vi "模拟量输入自动测试.vi"(8 "AD选择?":bool, 10 "DSP选择?":bool) -> ()   [LabVIEW 2010]
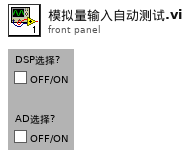
[diagram p1: front panel]
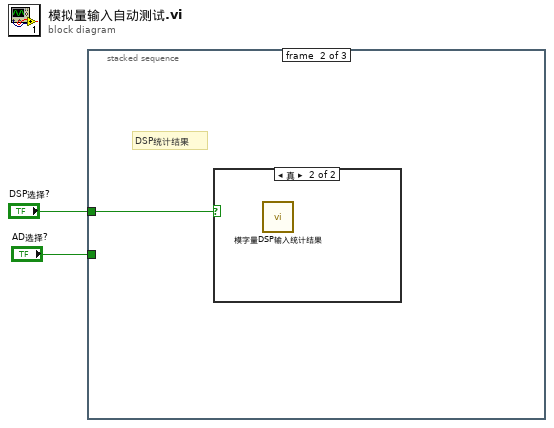
[diagram p0: block diagram]
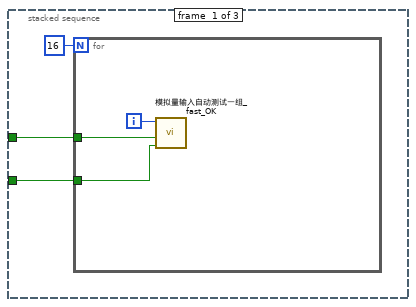
[diagram p2: hidden frame]
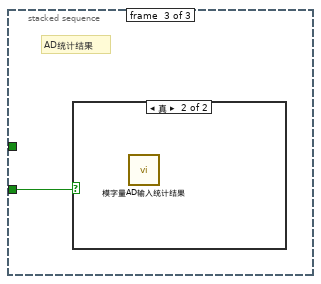
[diagram p4: hidden frame]
diagram:
  n1 = stacked-sequence {
    tunnel: "DSP选择?" -> [w4 w9 _]
    tunnel: "AD选择?" -> [w3 _ w10]
    frame #0 {
      n2 = for {
        N: 16 -> [_]
        tunnel: w4 -> [w7]
        tunnel: w3 -> [w6]
        i -> [w8]
        n3 = call "模拟量输入自动测试一组_fast_OK.vi"("AD选择？"=w6, "DSP选择？"=w7, "第几个"=w8) -> ()  [unwired: 9 in]
      }
    }
    frame #1 {
      # "DSP统计结果"
      n4 = case shown="真" w9 {
        frame False {
        }
        frame True {
          n5 = call "模字量DSP输入统计结果.vi"() -> ()  [unwired: 12 in]
        }
      }
    }
    frame #2 {
      # "AD统计结果"
      n6 = case shown="真" w10 {
        frame False {
        }
        frame True {
          n7 = call "模字量AD输入统计结果.vi"() -> ()  [unwired: 12 in]
        }
      }
    }
  }
